vi "Read initial setup.vi"(8 "error in (no error)":errorcluster, 11 "Channel in":refnum<class "Channel.lvclass">) -> (0 "error out":errorcluster, 3 "Channel out":refnum<class "Channel.lvclass">)   [LabVIEW 2018, in "Channel.lvclass"]
uses:
  Channel.lvclass
  Channel.lvclass/Channel.ctl
  <vilib>/Utility/config.llb/Read Key (U32).vi
  <vilib>/Utility/config.llb/Read Key (String).vi
  <vilib>/Utility/config.llb/NI_LVConfig.lvlib
panel:
  out "acs init configuration":T1={"Image path"=path "C:/images/today", "Remote IP"="200.131.64.25", "Channel"=1, "ACS mode"=0, "Communication"=0} {"Communication" items=["ZeroMQ", "TCP-IP"]; "ACS mode" items=["simulated", "real"]; "Channel" min=1 max=4}
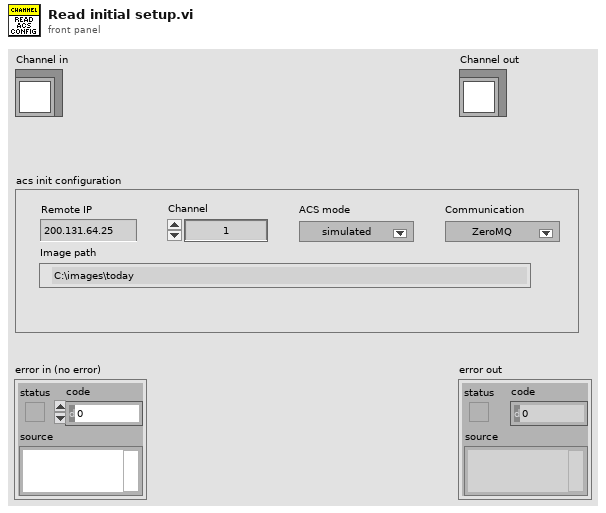
[diagram p1: front panel]
types:
  T1 = cluster{"Image path":path, "Remote IP":string, "Channel":u8, "ACS mode":u16, "Communication":u16}
  T2 = typedef "NI_LVConfig.lvlib/Config Data RefNum.ctl" = refnum<k1>
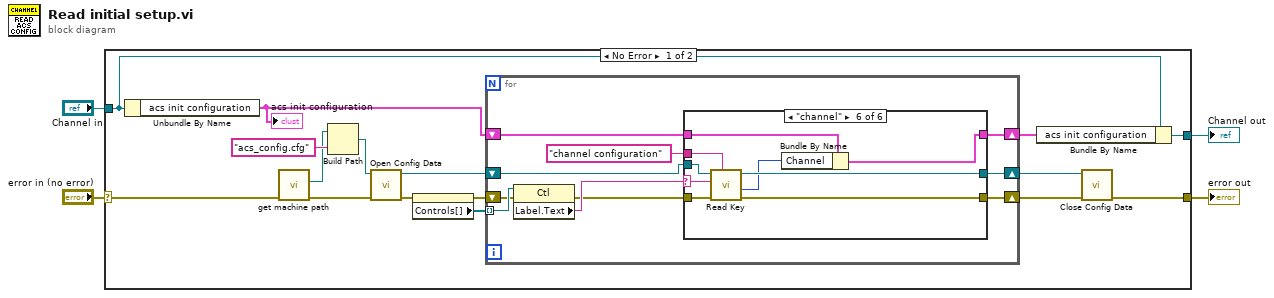
[diagram p0: block diagram]
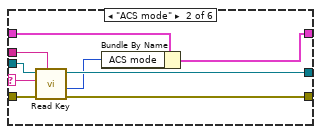
[diagram p3: hidden frame]
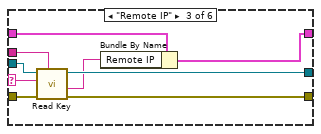
[diagram p4: hidden frame]
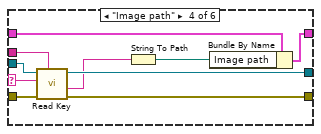
[diagram p5: hidden frame]
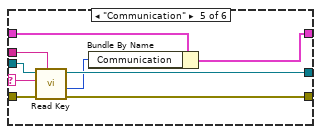
[diagram p6: hidden frame]
diagram:
  n1 = case shown="No Error" "error in (no error)" {
    selector: "error in (no error)" -> [w6 w81]
    tunnel: [w15 w81] -> w2
    tunnel: [w12 w80] -> w1
    tunnel: "Channel in" -> [w14 w80]
    frame No Error {
      n2 = Unbundle By Name(w14) -> ("acs init configuration"=w16:T1)
      "acs init configuration" <- w16
      n3 = call "get machine path.vi"("error in (no error) 2"=w6) -> ("error in (no error)"=w7:errorcluster, "machine path"=w5:path)  [unwired: 9 in]
      n4 = Build Path(base path=w5, name or relative path="acs_config.cfg") -> (appended path=w9:path)
      n5 = call <vilib>:"Open Config Data.vi"("error in (no error)"=w7, "configuration file path"=w9) -> ("error out"=w11:errorcluster, "refnum"=w18:T2)  [unwired: 7 in, 1 out]
      n6 = property on="acs init configuration" class="Clust (strict)"(error in=w11) -> (error out=w10:errorcluster, "Controls[]"=w20:refnum<vi>[])  [unwired: 1 in, 1 out]
      n7 = for {
        tunnel: w20 -> [w29] mode=indexing
        shift-right: [w27] -> w19
        shift-left: w10 -> [w25]
        shift-right: [w26] -> w17
        shift-left: w18 -> [w24]
        shift-right: [w22] -> w13
        shift-left: w16 -> [w30]
        n8 = property class="Ctl"(reference=w29, error in=w25) -> (error out=w23:errorcluster, "Label.Text"=w28:string)  [unwired: 1 out]
        n9 = case shown="\"channel\"" w28 {
          selector: w28 -> [_ w40 w49 w59 w68 w77]
          tunnel: [w32 w41 w50 w60 w69 w78] -> w26
          tunnel: [w31 w42 w51 w61 w70 w79] -> w27
          tunnel: w30 -> [w33 w38 w47 w56 w66 w75]
          tunnel: [w33 w37 w46 w55 w65 w74] -> w22
          tunnel: w24 -> [w32 w35 w45 w53 w64 w73]
          tunnel: w23 -> [w31 w34 w44 w52 w63 w72]
          tunnel: "channel configuration" -> [_ w36 w43 w54 w62 w71]
          frame "False", Default {
          }
          frame "ACS mode" {
            n10 = call-poly <vilib>:"Read Key.vi"("section"=w36, "error in (no error)"=w34, "key"=w40, "refnum"=w35) -> ("error out"=w42:errorcluster, "value"=w39:u32, "refnum out"=w41:T2)  [unwired: 4 in, 1 out]
            n11 = Bundle By Name(cluster=w38, "ACS mode"=w39) -> (w37:T1)
          }
          frame "Remote IP" {
            n12 = call-poly <vilib>:"Read Key.vi"("section"=w43, "error in (no error)"=w44, "key"=w49, "refnum"=w45) -> ("error out"=w51:errorcluster, "value"=w48:string, "refnum out"=w50:T2)  [unwired: 4 in, 1 out]
            n13 = Bundle By Name(cluster=w47, "Remote IP"=w48) -> (w46:T1)
          }
          frame "Image path" {
            n14 = call-poly <vilib>:"Read Key.vi"("section"=w54, "error in (no error)"=w52, "key"=w59, "refnum"=w53) -> ("error out"=w61:errorcluster, "value"=w57:string, "refnum out"=w60:T2)  [unwired: 4 in, 1 out]
            n15 = String To Path(string=w57) -> (path=w58:path)
            n16 = Bundle By Name(cluster=w56, "Image path"=w58) -> (w55:T1)
          }
          frame "Communication" {
            n17 = call-poly <vilib>:"Read Key.vi"("section"=w62, "error in (no error)"=w63, "key"=w68, "refnum"=w64) -> ("error out"=w70:errorcluster, "value"=w67:u32, "refnum out"=w69:T2)  [unwired: 4 in, 1 out]
            n18 = Bundle By Name(cluster=w66, "Communication"=w67) -> (w65:T1)
          }
          frame "channel" {
            n19 = call-poly <vilib>:"Read Key.vi"("section"=w71, "error in (no error)"=w72, "key"=w77, "refnum"=w73) -> ("error out"=w79:errorcluster, "value"=w76:u32, "refnum out"=w78:T2)  [unwired: 4 in, 1 out]
            n20 = Bundle By Name(cluster=w75, "Channel"=w76) -> (w74:T1)
          }
        }
      }
      n21 = Bundle By Name(cluster=w14, "acs init configuration"=w13) -> (w12:refnum<class "Channel.lvclass">)
      n22 = call <vilib>:"Close Config Data.vi"("error in (no error)"=w19, "refnum"=w17) -> ("error out"=w15:errorcluster)  [unwired: 8 in, 1 out]
    }
    frame Error {
    }
  }
  "error out" <- w2
  "Channel out" <- w1
